vi "Operator Dialog.vi"(11 "Message":string="Create Bench Ref") -> ()   [LabVIEW 2024, in "BenchParent.lvclass"]
uses:
  BenchParent.lvclass
  BenchParent.lvclass/BenchParent.ctl
panel:
  out "Display":string
  in  "Boolean":bool
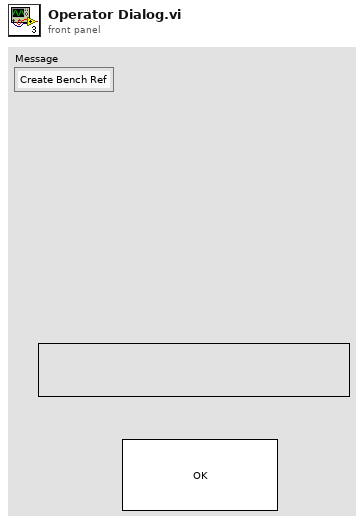
[diagram p1: front panel]
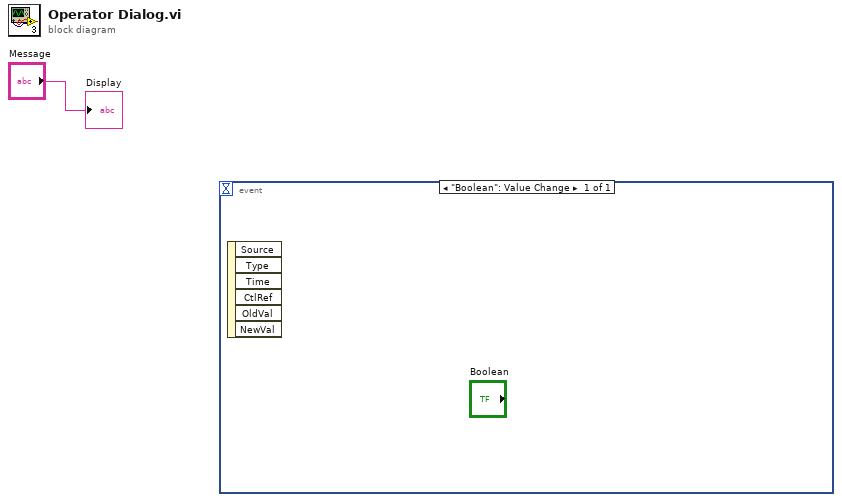
[diagram p0: block diagram]
diagram:
  n1 = event shown="[0] \"Boolean\": Value Change" {
    selector: _ -> [_]
    dyn-events: _ -> [_]
    timeout: _ -> [_]
    event "Boolean": Value Change {
      n2 = event-data() -> ()  [unwired: 1 in, 6 out]
    }
  }
  "Display" <- "Message"
